vi "Keithley 27XX Continuous Multi Read.vi"() -> ()   [LabVIEW 2020]
doc: "This example VI shows how to take a measurement continuously."
uses:
  <instrlib>/Keithley 27XX/Public/Data/Read Data Buffer Subset.vi
  <instrlib>/Keithley 27XX/Keithley 27XX.lvlib
panel:
  in  "Serial Configuration":T1={"Baud Rate (9600)"=9600, "Flow Control (1: XON/XOFF)"=1, "Termination Char (0:CR)"=0} {"Termination Char (0:CR)" items=["CR", "LF"]; "Flow Control (1: XON/XOFF)" items=["None", "XON/XOFF", "RTS/CTS (2701 Only)", "XON/XOFF & RTS/CTS (2701 Only)"]; "Baud Rate (9600)" items=["300"=300, "600"=600, "1200"=1200, "2400"=2400, "4800"=4800, "9600"=9600, "19.2k"=19200, "38.4k (2701 Only)"=38400, "57.6k (2701 Only)"=57600, "115.2k (2701 Only)"=115200]}
  out "Measurement Data":dbl[](array[numeric])
  in  "Stop":bool
  in  "Function (0: DC Voltage)":u16(ring) items=["DC Voltage", "AC Voltage", "DC Current", "AC Current", "Resistance", "Four-Wire Resistance", "Temperature (C)", "Frequency", "Period", "Continuity"]
  in  "Channel List (101:110)":string="101:110"
  in  "VISA resource name":refnum<visa-resource-name>
  # "© 2005 National Instruments Corporation.  ALL RIGHTS RESERVED."
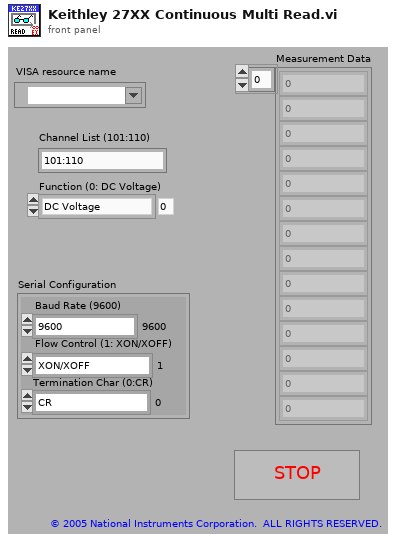
[diagram p1: front panel]
types:
  T1 = cluster{"Baud Rate (9600)":u32, "Flow Control (1: XON/XOFF)":u16, "Termination Char (0:CR)":u16}
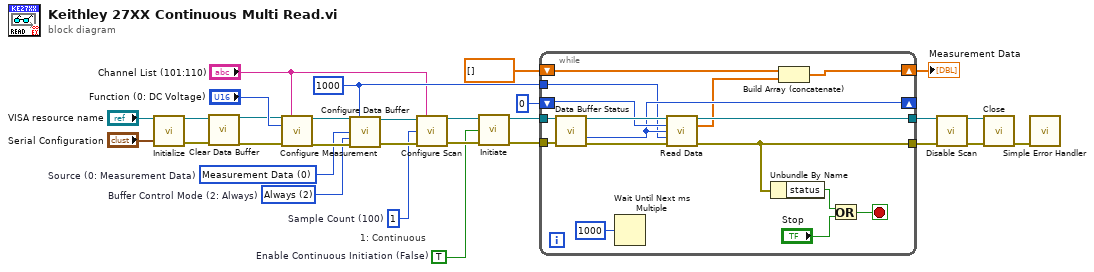
[diagram p0: block diagram]
diagram:
  w6 = TRUE  # Enable Continuous Initiation (False)
  w8 = 1  # Sample Count (100)
  w22 = u16 0 items=["Measurement Data", "Math Data", "None"]  # Source (0: Measurement Data)
  w19 = 1000 ("Buffer Size (100)")
  w21 = u16 2 items=["Never", "Next", "Always"]  # Buffer Control Mode (2: Always)
  # "1: Continuous"
  n1 = call <instrlib>:"Initialize.vi"("VISA resource name"="VISA resource name", "Serial Configuration"="Serial Configuration") -> ("VISA resource name out"=w2:refnum<visa-resource-name>, "error out"=w3:errorcluster)  [unwired: 12 in]
  n2 = call <instrlib>:"Clear Data Buffer.vi"("VISA resource name"=w2, "error in (no error)"=w3) -> ("VISA resource name out"=w5:refnum<visa-resource-name>, "error out"=w4:errorcluster)  [unwired: 12 in]
  n3 = call <instrlib>:"Configure Measurement.vi"("VISA resource name"=w5, "Scan List (Empty)"="Channel List (101:110)", "Function (0: DC Voltage)"="Function (0: DC Voltage)", "error in (no error)"=w4) -> ("VISA resource name out"=w26:refnum<visa-resource-name>, "error out"=w25:errorcluster)  [unwired: 10 in]
  n4 = call <instrlib>:"Configure Data Buffer.vi"("VISA resource name"=w26, "Buffer Size (1000)"=w19, "Source (0: Measurement Data)"=w22, "Buffer Control Mode (2: Always)"=w21, "error in (no error)"=w25) -> ("VISA resource name out"=w24:refnum<visa-resource-name>, "error out"=w23:errorcluster)  [unwired: 9 in]
  n5 = call <instrlib>:"Configure Scan.vi"("VISA resource name"=w24, "Channel List (101:110)"="Channel List (101:110)", "Sample Count (100)"=w8, "error in (no error)"=w23) -> ("VISA resource name out"=w18:refnum<visa-resource-name>, "error out"=w17:errorcluster)  [unwired: 10 in]
  n6 = call <instrlib>:"Initiate.vi"("VISA resource name"=w18, "Enable Continuous Initiation (False)"=w6, "error in (no error)"=w17) -> ("VISA resource name out"=w15:refnum<visa-resource-name>, "error out"=w16:errorcluster)  [unwired: 11 in]
  n7 = while {
    tunnel: [w44] -> w11
    tunnel: [w39] -> w14
    shift-right: [w40] -> w7
    shift-left: dbl[] [] -> [w45]
    shift-right: [w32] -> _
    shift-left: 0 -> [w33]
    tunnel: w19 -> [w31]
    tunnel: w16 -> [w35]
    tunnel: w15 -> [w34]
    stop <- w36 stop-if-true
    n8 = call <instrlib>:"Data Buffer Status.vi"("VISA resource name"=w34, "error in (no error)"=w35) -> ("VISA resource name out"=w43:refnum<visa-resource-name>, "Next Buffer Location"=w32:i32, "error out"=w42:errorcluster)  [unwired: 9 in, 2 out]
    n9 = Wait Until Next ms Multiple(millisecond multiple=u32 1000 ("milliseconds to wait")) -> ()  [unwired: 1 out]
    n10 = call-poly <instrlib>:"Read Data.vi"("VISA resource name"=w43, "Previous Buffer Read Location (0)"=w33, "Next Buffer Location (0)"=w32, "Buffer Size (1000)"=w31, "error in (no error)"=w42) -> ("VISA resource name out"=w44:refnum<visa-resource-name>, "Measurement Data"=w30:dbl[], "error out"=w39:errorcluster)  [unwired: 5 in, 3 out]
    n11 = Unbundle By Name(w39) -> ("status"=w37:bool)
    n12 = Build Array (concatenate)(w45, w30) -> (w40:dbl[])
    n13 = Or(x=w37, y="Stop") -> (x .or. y?=w36:bool)
  }
  "Measurement Data" <- w7
  n14 = call <instrlib>:"Disable Scan.vi"("VISA resource name"=w11, "error in (no error)"=w14) -> ("VISA resource name out"=w12:refnum<visa-resource-name>, "error out"=w13:errorcluster)  [unwired: 12 in]
  n15 = call <instrlib>:"Close.vi"("VISA resource name"=w12, "error in (no error)"=w13) -> ("error out"=w10:errorcluster)  [unwired: 13 in]
  n16 = call <vilib>:"Simple Error Handler.vi"("error in (no error)"=w10) -> ()  [unwired: 4 in, 5 out]
